vi "Object_Set Attributes.vi"(8 "error in (no error)":errorcluster, 10 "Object Attributes":T1, 11 "GObject in":refnum<class "Object.lvclass">) -> (0 "error out":errorcluster, 3 "GObject out":refnum<class "Object.lvclass">)   [LabVIEW 2017, in "Front Panel Publisher.lvlib" / "Object.lvclass"]
uses:
  Object.lvclass
  Coordinates.ctl
  Attributes.ctl
  <vilib>/Utility/miscctls.llb/LVRectTypeDef.ctl
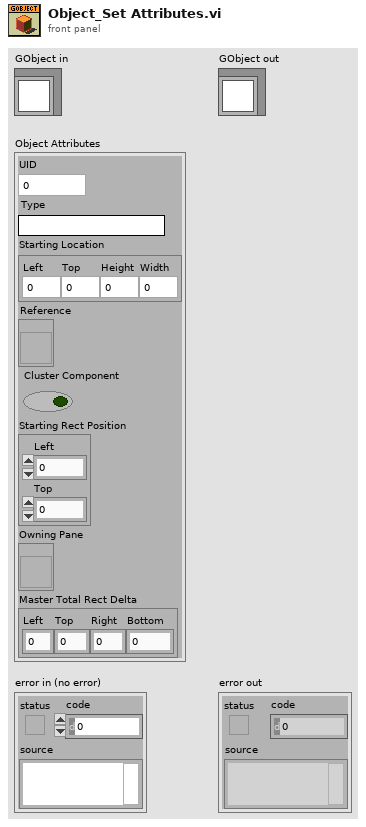
[diagram p1: front panel]
types:
  T1 = typedef "Front Panel Publisher.lvlib/Object.lvclass/Attributes.ctl" = cluster{"UID":i32, "Type":string, "Starting Location":T2, "Reference":refnum<vi>, "Cluster Component":bool, "Starting Rect Position":cluster{"Left":i16, "Top":i16}, "Owning Pane":refnum<vi>, "Master Total Rect Delta":T3}
  T2 = typedef "Front Panel Publisher.lvlib/Object.lvclass/Coordinates.ctl" = cluster{"Left":i32, "Top":i32, "Height":u32, "Width":u32}
  T3 = typedef "LVRectTypeDef.ctl" = cluster{"Left":i16, "Top":i16, "Right":i16, "Bottom":i16}
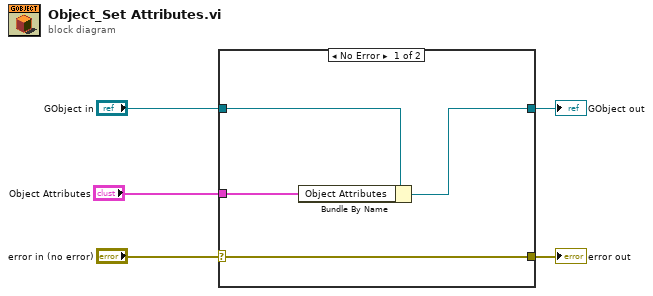
[diagram p0: block diagram]
diagram:
  n1 = case shown="No Error" "error in (no error)" {
    selector: "error in (no error)" -> [w8 w11]
    tunnel: [w8 w11] -> w4
    tunnel: [w7 w10] -> w2
    tunnel: "GObject in" -> [w9 w10]
    tunnel: "Object Attributes" -> [w6 _]
    frame No Error {
      n2 = Bundle By Name(cluster=w9, "Object Attributes"=w6) -> (w7:refnum<class "Object.lvclass">)
    }
    frame Error {
    }
  }
  "error out" <- w4
  "GObject out" <- w2
